vi "Get_USER_ID.vi"(8 "错误输入":errorcluster, 11 "USER_EMPLOYEE_ID":string) -> (0 "错误输出":errorcluster, 3 "USER_ID":string)   [LabVIEW 2020]
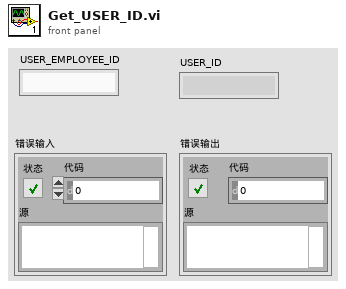
[diagram p1: front panel]
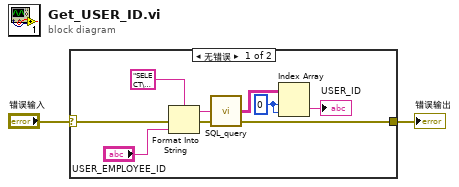
[diagram p0: block diagram]
diagram:
  n1 = case shown="无错误" "错误输入" {
    selector: "错误输入" -> [w8 w12]
    tunnel: [w6 w12] -> w1
    frame No Error {
      w10 = 0 ("索引 (行)")
      n2 = Format Into String(format string="SELECT\ndbo.[User].USER_ID\n\nFROM\ndbo.[User]\nWHERE\ndbo.[User].USER_EMPLOYEE_ID = '%s'\n", error in=w8, "USER_EMPLOYEE_ID") -> (resulting string=w11:string, error out=w7:errorcluster)  [unwired: 1 in]
      n3 = call "SQL_query.vi"("error in (no error)"=w7, "SQL query"=w11) -> ("error out"=w6:errorcluster, "data"=w5:string[][])  [unwired: 1 in, 1 out]
      n4 = Index Array(array=w5, index (row)=w10, index (col)=w10) -> (element=→"USER_ID":string)
    }
    frame Error {
    }
  }
  "错误输出" <- w1
